vi "Create from Info.vi"(8 "error in (no error)":errorcluster, 9 "Folder":path, 10 "Package Info":T1, 11 "GitPackageAbstract in":refnum<class "GitPackage.lvclass">) -> (0 "error out":errorcluster, 3 "GitPackageAbstract out":refnum<class "GitPackage.lvclass">)   [LabVIEW 2020, in "GPack.lvlib" / "GitPackage.lvclass"]
uses:
  GitPackage.lvclass
  Package Info.ctl
  GitPackage.lvclass/GitPackage.ctl
  GPack.lvlib
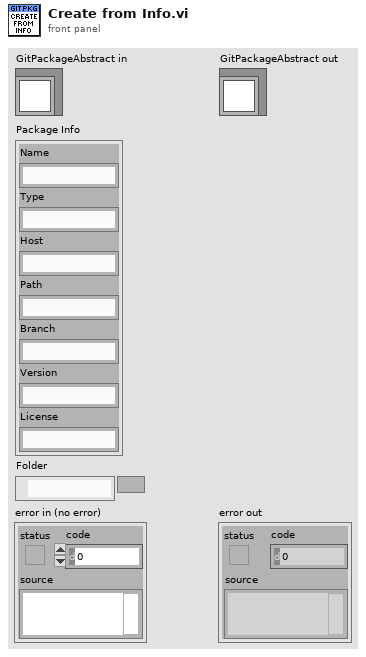
[diagram p1: front panel]
types:
  T1 = typedef "GPack.lvlib/Package Info.ctl" = cluster{"Name":string, "Type":string, "Host":string, "Path":string, "Branch":string, "Version":string, "License":string}
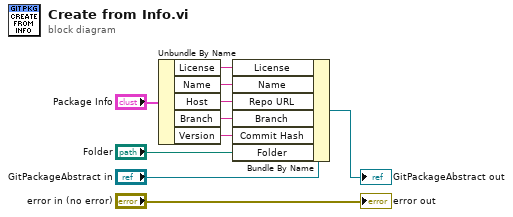
[diagram p0: block diagram]
diagram:
  n1 = Unbundle By Name("Package Info") -> ("License"=w1:string, "Name"=w3:string, "Host"=w4:string, "Branch"=w5:string, "Version"=w6:string)
  n2 = Bundle By Name(cluster="GitPackageAbstract in", "License"=w1, "Name"=w3, "Repo URL"=w4, "Branch"=w5, "Commit Hash"=w6, "Folder"="Folder") -> (→"GitPackageAbstract out":refnum<class "GitPackage.lvclass">)
  "error out" <- "error in (no error)"
